vi "FormatPath.vi"(0 "Path":path, 1 "type":T1) -> (2 "value":string)   [LabVIEW 2014, in "PythonConfiguration.lvclass"]
uses:
  PythonConfiguration.lvclass
  TypeDefs/PathTypeTD.ctl
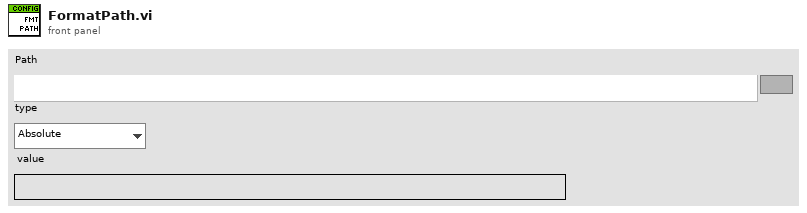
[diagram p1: front panel]
types:
  T1 = typedef "PythonConfiguration.lvclass/PathTypeTD.ctl" = enum16{"Absolute", "Relative to Config", "Relative to App"}
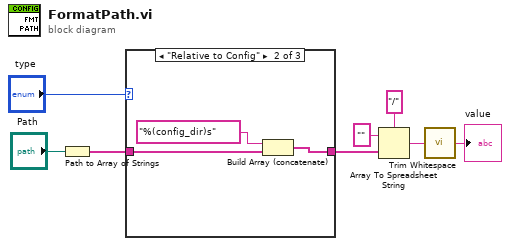
[diagram p0: block diagram]
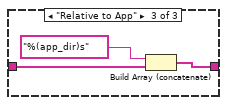
[diagram p3: hidden frame]
diagram:
  n1 = Path to Array of Strings(0:"Path") -> (2:w6:string[])  [unwired: 1 out]
  n2 = case shown="\"Relative to Config\"" "type" {
    tunnel: w6 -> [w9 w12 w15]
    tunnel: [w9 w10 w13] -> w5
    frame "Absolute" {
    }
    frame "Relative to Config" {
      n3 = Build Array (concatenate)("%(config_dir)s", w12) -> (w10:string[])
    }
    frame "Relative to App" {
      n4 = Build Array (concatenate)("%(app_dir)s", w15) -> (w13:string[])
    }
  }
  n5 = Array To Spreadsheet String(delimiter (Tab)="/", array=w5, 3:"" ("format string")) -> (spreadsheet string=w2:string)
  n6 = call <vilib>:"Trim Whitespace.vi"("string"=w2) -> ("trimmed string"=→"value":string)  [unwired: 1 in]
